vi "Read Output.vi"(8 "error in (no error)":errorcluster, 10 "Channel (0: 30V Channel)":T1 caption="Channel (0: +6V)" items=["30V/3A Channel", "30V/3A Channel", "5V/3A Channel"], 11 "VISA resource name":refnum<visa-resource-name>) -> (0 "error out":errorcluster, 1 "Actual Current Level (A)":dbl caption="Actual Current Level" format="%.2f", 2 "Actual Voltage Level (V)":dbl caption="Actual Voltage Level" format="%.2f", 3 "VISA resource name out":refnum<visa-resource-name>, 5 "Actual Power Level (W)":dbl caption="Actual Power Level" format="%.2f")   [LabVIEW 2020, in "Library Instrument & Equipement.lvlib" / "Library Power_Supply.lvlib" / "RIGOL DP800 Series.lvlib"]
doc: "Returns the actual voltage level and actual current level for a desired channel."
uses:
  RIGOL DP800 Series.lvlib
  Channels.ctl
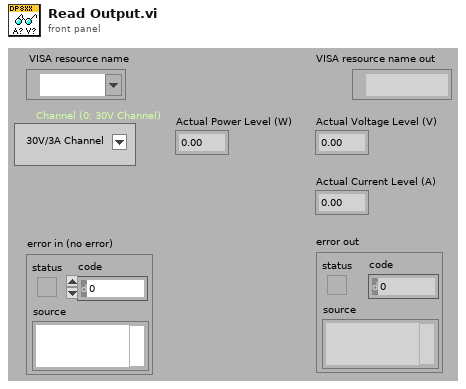
[diagram p1: front panel]
types:
  T1 = typedef "Library Instrument & Equipement.lvlib/Library Power_Supply.lvlib/RIGOL DP800 Series.lvlib/Channels.ctl" = i32
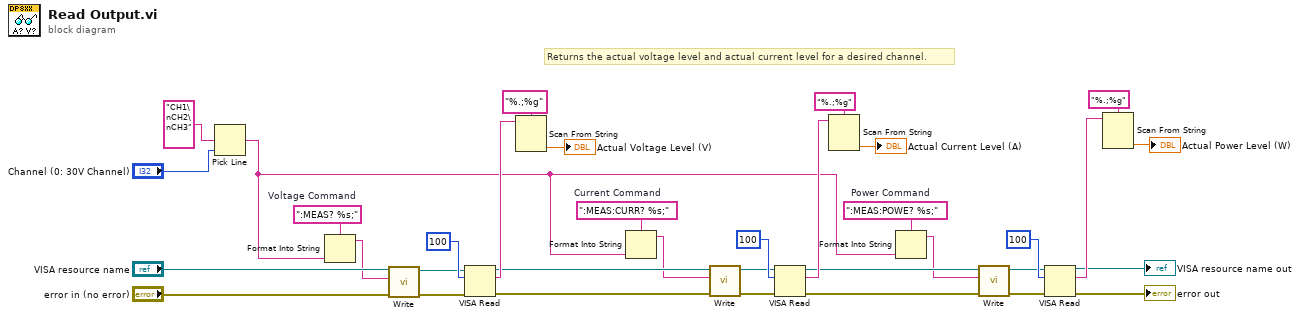
[diagram p0: block diagram]
diagram:
  w22 = ":MEAS:POWE? %s;"  # Power Command
  w24 = ":MEAS:CURR? %s;"  # Current Command
  w25 = ":MEAS? %s;"  # Voltage Command
  # "Returns the actual voltage level and actual current level for a desired channel."
  n1 = Pick Line(multi-line string="CH1\nCH2\nCH3", line index="Channel (0: 30V Channel)") -> (output string=w21:string)  [unwired: 1 in]
  n2 = Format Into String(format string=w25, w21) -> (resulting string=w11:string)  [unwired: 2 in, 1 out]
  n3 = call "Write.vi"("error in (no error)"="error in (no error)", "Write Buffer (\"\")"=w11, "VISA resource name"="VISA resource name") -> ("error out"=w15:errorcluster, "VISA resource name out"=w14:refnum<visa-resource-name>)  [unwired: 7 in]
  n4 = VISA Read(VISA resource name=w14, byte count=u32 100, error in (no error)=w15) -> (VISA resource name out=w7:refnum<visa-resource-name>, read buffer=w34:string, error out=w8:errorcluster)  [unwired: 1 out]
  n5 = Scan From String(format string="%.;%g", input string=w34) -> (output 1=→"Actual Voltage Level (V)":dbl)  [unwired: 3 in, 3 out]
  n6 = Format Into String(format string=w24, w21) -> (resulting string=w6:string)  [unwired: 2 in, 1 out]
  n7 = call "Write.vi"("error in (no error)"=w8, "Write Buffer (\"\")"=w6, "VISA resource name"=w7) -> ("error out"=w9:errorcluster, "VISA resource name out"=w10:refnum<visa-resource-name>)  [unwired: 7 in]
  n8 = VISA Read(VISA resource name=w10, byte count=u32 100, error in (no error)=w9) -> (VISA resource name out=w3:refnum<visa-resource-name>, read buffer=w31:string, error out=w4:errorcluster)  [unwired: 1 out]
  n9 = Scan From String(format string="%.;%g", input string=w31) -> (output 1=→"Actual Current Level (A)":dbl)  [unwired: 3 in, 3 out]
  n10 = Format Into String(format string=w22, w21) -> (resulting string=w1:string)  [unwired: 2 in, 1 out]
  n11 = call "Write.vi"("error in (no error)"=w4, "Write Buffer (\"\")"=w1, "VISA resource name"=w3) -> ("error out"=w5:errorcluster, "VISA resource name out"=w2:refnum<visa-resource-name>)  [unwired: 7 in]
  n12 = VISA Read(VISA resource name=w2, byte count=u32 100, error in (no error)=w5) -> (VISA resource name out=→"VISA resource name out":refnum<visa-resource-name>, read buffer=w19:string, error out=→"error out":errorcluster)  [unwired: 1 out]
  n13 = Scan From String(format string="%.;%g", input string=w19) -> (output 1=→"Actual Power Level (W)":dbl)  [unwired: 3 in, 3 out]
